vi "Analyze State from Event.vi"(8 "error in (no error)":errorcluster, 10 "Debug Data.lvclass":refnum<class "Debug Data.lvclass">, 11 "Debugger In":refnum<class "Debugger.lvclass">) -> (0 "error out":errorcluster, 3 "Debugger Out":refnum<class "Debugger.lvclass">)   [LabVIEW 2020, in "Debugger.lvclass"]
uses:
  Debugger.lvclass
  Debug Data/Debug Data.lvclass
  Debugger.lvclass/Debugger.ctl
  State Analyzer/Debug State Analyzer.lvclass
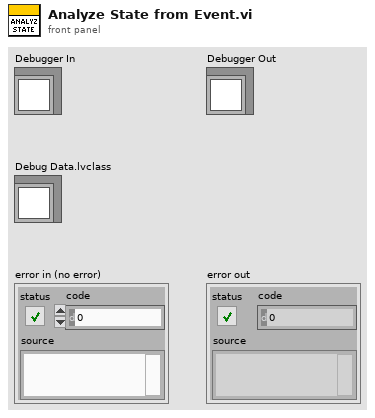
[diagram p1: front panel]
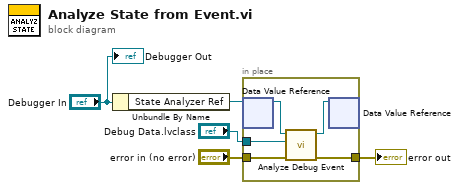
[diagram p0: block diagram]
diagram:
  n1 = Unbundle By Name("Debugger In") -> ("State Analyzer Ref"=w1:refnum<data-value>)
  n2 = in-place {
    in-place-border: "Debug Data.lvclass" -> [w10]
    in-place-border: [w9] -> w3
    in-place-border: "error in (no error)" -> [w8]
    n3 = in-place-dvr #1(w1) -> (w7:refnum<class "Debug State Analyzer.lvclass">)  [unwired: 1 out]
    n4 = call "Analyze Debug Event.vi"("error in (no error)"=w8, "Debug Data.lvclass"=w10, "Debug State Analyzer In"=w7) -> ("error out"=w9:errorcluster, "Debug State Analyzer Out"=w6:refnum<class "Debug State Analyzer.lvclass">)  [unwired: 7 in]
    n5 = in-place-dvr #1(w6) -> ()  [unwired: 2 out]
  }
  "error out" <- w3
  "Debugger Out" <- "Debugger In"
